vi "HEWH Intellifaucet Temp Equation.vi"(8 "Error In":errorcluster, 11 "Temp/GPM Target":dbl) -> (0 "Error Out":errorcluster, 3 "Temp uA":i32)   [LabVIEW 2016]
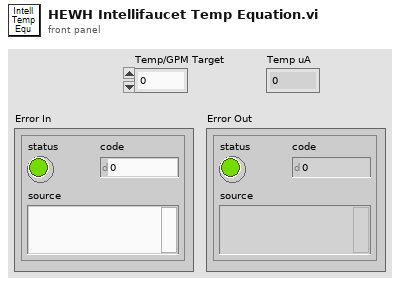
[diagram p1: front panel]
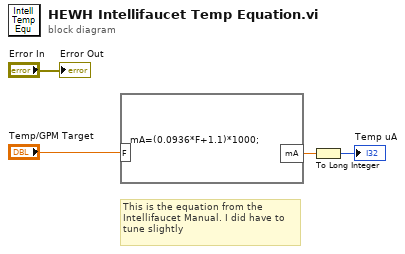
[diagram p0: block diagram]
diagram:
  # "This is the equation from the \nIntellifaucet Manual. I did have to\ntune slightly"
  n1 = formula code="mA=(0.0936*F+1.1)*1000;"("F"="Temp/GPM Target") -> ("mA"=w3:dbl)
  n2 = To Long Integer(number=w3) -> (32bit integer=→"Temp uA":i32)
  "Error Out" <- "Error In"
